vi "Contionue Case Update Output Table.vi"() -> (0 "error out":errorcluster)   [LabVIEW 2023, in "HardwareAbstractionLayer_LVOOP.lvlib" / "Report.lvclass"]
uses:
  Database/SQL Public VI/Control/DB Options.ctl
  <vilib>/Utility/error.llb/Trim Whitespace One-Sided.vi
  Report.lvclass
  Report.lvclass/Report.ctl
  Database/Database.lvclass
  Control/Result FGV Data.ctl
  Control/Action FGV.ctl
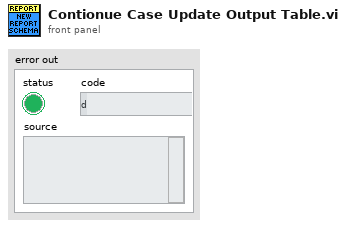
[diagram p1: front panel]
types:
  T1 = typedef "HardwareAbstractionLayer_LVOOP.lvlib/Database.lvclass/DB Options.ctl" = enum16{"Init", "Select Data", "Insert Data", "Update Data", "Delete Data", "Execute Query", "Create Schema", "Create Table", "List Tables", "List Columns", "Close"}
  T2 = typedef "HardwareAbstractionLayer_LVOOP.lvlib/Report.lvclass/Result FGV Data.ctl" = cluster{"Project Name":string, "Product Name":string, "Product Varient":string, "Test Name":string, "Test Phase":string, "Test Description":string, "Temp Chamber Name":string, "Schema":string, "Total No of Cycles":u32, "Current Cycle Number":u32, "Cycle Duration":u32, "Current Test Mode":string}
  T3 = typedef "HardwareAbstractionLayer_LVOOP.lvlib/Report.lvclass/Action FGV.ctl" = enum16{"Init", "Set Project Name", "Set Product Name", "Set Product Varient", "Set Test Name", "Set Test Phase", "Set Test Description", "Set Temp Chamber Name", "Set Cycle Duration", "Set Current Cycle Number", "Set Schema", "Set Total No Of Cycle", "Set Current Test Mode", "Set All Data", "Get All Data"}
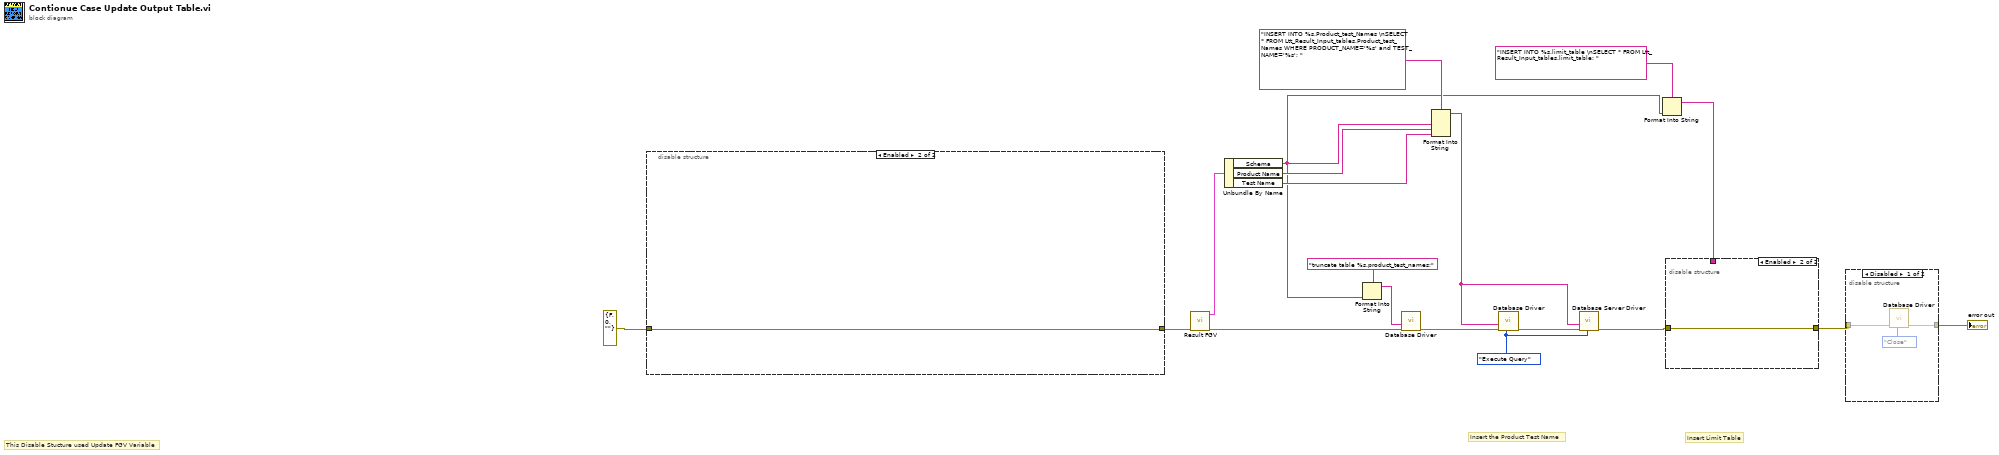
[diagram p0: block diagram]
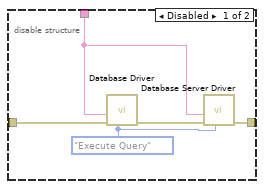
[diagram p2: hidden frame]
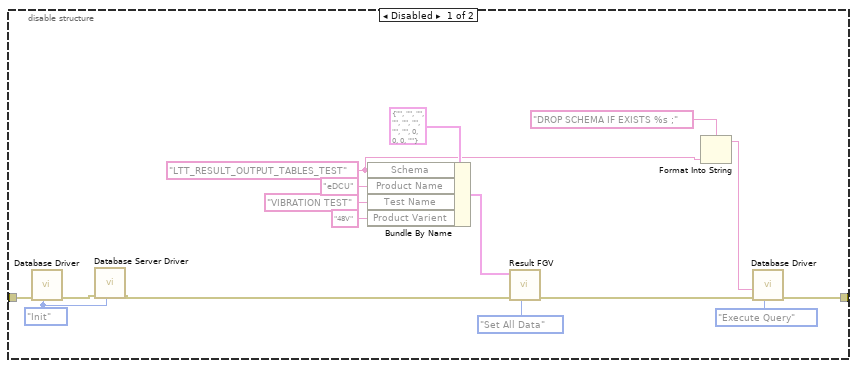
[diagram p3: hidden frame]
diagram:
  w9 = DB_Options."Execute Query" ("Options")
  # "Insert Limit Table"
  # "This Disable Stucture used Update FGV Variable"
  # "Insert the Product Test Name"
  n1 = disable-structure shown="Enabled" {
    disable-tunnel: errorcluster {"status"=FALSE, "code"=0, "source"=""} ("error in") -> [w35 w36]
    disable-tunnel: [w34 w36] -> w14
    frame Disabled {
      w21 = DB_Options."Init" ("Options")
      w23 = "LTT_RESULT_OUTPUT_TABLES_TEST" ("Schema")
      n2 = call "Database Driver.vi"("Options"=w21, "error in"=w35) -> ("error out"=w22:errorcluster)  [unwired: 6 in, 3 out]
      n3 = call "Database Server Driver.vi"("Options"=w21, "error in"=w22) -> ("error out"=w20:errorcluster)  [unwired: 6 in, 3 out]
      n4 = Bundle By Name(cluster=T2 {"Project Name"="", "Product Name"="", "Product Varient"="", "Test Name"="", "Test Phase"="", "Test Description"="", "Temp Chamber Name"="", "Schema"="", "Total No of Cycles"=0, "Current Cycle Number"=0, "Cycle Duration"=0, "Current Test Mode"=""} ("Result FGV Data In"), "Schema"=w23, "Product Name"="eDCU", "Test Name"="VIBRATION TEST", "Product Varient"="48V") -> (w31:T2)
      n5 = call "Result FGV.vi"("Action(Get All Data)"=Action_FGV."Set All Data" ("Action"), "error in"=w20, "Result FGV Data In"=w31) -> ("error out"=w27:errorcluster)  [unwired: 7 in, 1 out]
      n6 = Format Into String(format string="DROP SCHEMA IF EXISTS %s ;", w23) -> (resulting string=w24:string)  [unwired: 2 in, 1 out]
      n7 = call "Database Driver.vi"("Options"=DB_Options."Execute Query", "error in"=w27, "SQL query"=w24) -> ("error out"=w34:errorcluster)  [unwired: 5 in, 3 out]
    }
    frame Enabled {
    }
  }
  n8 = call "Result FGV.vi"("error in"=w14) -> ("error out"=w6:errorcluster, "Result FGV Data Out"=w18:T2)  [unwired: 9 in]
  n9 = Unbundle By Name(w18) -> ("Schema"=w1:string, "Product Name"=w13:string, "Test Name"=w2:string)
  n10 = Format Into String(format string="truncate table %s.product_test_names;", w1) -> (resulting string=w4:string)  [unwired: 2 in, 1 out]
  n11 = call "Database Driver.vi"("error in"=w6, "SQL query"=w4) -> ("error out"=w5:errorcluster)  [unwired: 6 in, 3 out]
  n12 = Format Into String(format string="INSERT INTO %s.Product_test_Names \nSELECT * FROM Ltt_Result_Input_tables.Product_test_Names WHERE PRODUCT_NAME='%s' and TEST_NAME='%s'; ", w1, w13, w2) -> (resulting string=w10:string)  [unwired: 2 in, 1 out]
  n13 = call "Database Driver.vi"("Options"=w9, "error in"=w5, "SQL query"=w10) -> ("error out"=w12:errorcluster)  [unwired: 5 in, 3 out]
  n14 = call "Database Server Driver.vi"("Options"=w9, "error in"=w12, "SQL query"=w10) -> ("error out"=w11:errorcluster)  [unwired: 5 in, 3 out]
  n15 = Format Into String(format string="INSERT INTO %s.limit_table \nSELECT * FROM Ltt_Result_Input_tables.limit_table; ", w1) -> (resulting string=w7:string)  [unwired: 2 in, 1 out]
  n16 = disable-structure shown="Enabled" {
    disable-tunnel: w11 -> [w41 w42]
    disable-tunnel: [w39 w42] -> w8
    disable-tunnel: w7 -> [w37 _]
    frame Disabled {
      w38 = DB_Options."Execute Query" ("Options")
      n17 = call "Database Driver.vi"("Options"=w38, "error in"=w41, "SQL query"=w37) -> ("error out"=w40:errorcluster)  [unwired: 5 in, 3 out]
      n18 = call "Database Server Driver.vi"("Options"=w38, "error in"=w40, "SQL query"=w37) -> ("error out"=w39:errorcluster)  [unwired: 5 in, 3 out]
    }
    frame Enabled {
    }
  }
  n19 = disable-structure shown="Disabled" {
    disable-tunnel: [w44 w46] -> w19
    disable-tunnel: w8 -> [w43 w46]
    frame Disabled {
      n20 = call "Database Driver.vi"("Options"=DB_Options."Close", "error in"=w43) -> ("error out"=w44:errorcluster)  [unwired: 6 in, 3 out]
    }
    frame Enabled {
    }
  }
  "error out" <- w19
